vi "Test2_R_S.vi"() -> ()   [LabVIEW 2023, in "R_S.lvlib"]
uses:
  R_S.lvlib
panel:
  out "error out":errorcluster
  in  "VISA_CMD":string="SYST:PRES"
  in  "VISA in":refnum<visa-resource-name>="TCPIP::Vince_Wu-NB::inst0::INSTR"
  # "SG IP : TCPIP::192.168.88.12::hislip0::INSTR\nSA IP :  TCPIP::Vince_Wu-NB::inst0::INSTR"
  # "TCPIP::Vince_Wu-NB::inst0::INSTR"
  # "*IDN?"
  # "FETCh:WLAN:MEAS:MEValuation:TRACe:EVMagnitude:SYMBol:AVERage?"
  # "SYST:ERR?"
  # "SOUR:GPRF:GEN:RFS:LEV -20"
  # "FETCh:BURSt:ALL:FORMatted?"
  # "FETCh:BURSt:PPDU:EVM:ALL:AVERage?\nFETCh:WLAN:MEAS:MEValuation:TRACe:EVMagnitude:SYMBol:AVERage?"
  # "FETCh:BURSt:PPDU:EVM:ALL:AVERage?"
  # "FETC:BURS:ALL:FORM?"
  # "FETCh:BURSt:ALL:FORMatted?"
  # "setSA\nINIT:BLOC:CONT OFF,'Group 1'\nINIT:BLOC:IMM\nDISP:TRAC:Y:RLEV -10dBm"
  # "setPower\nSOUR:GPRF:GEN:RFS:LEV -15\n\nSOUR:GPRF:GEN:STAT ON"
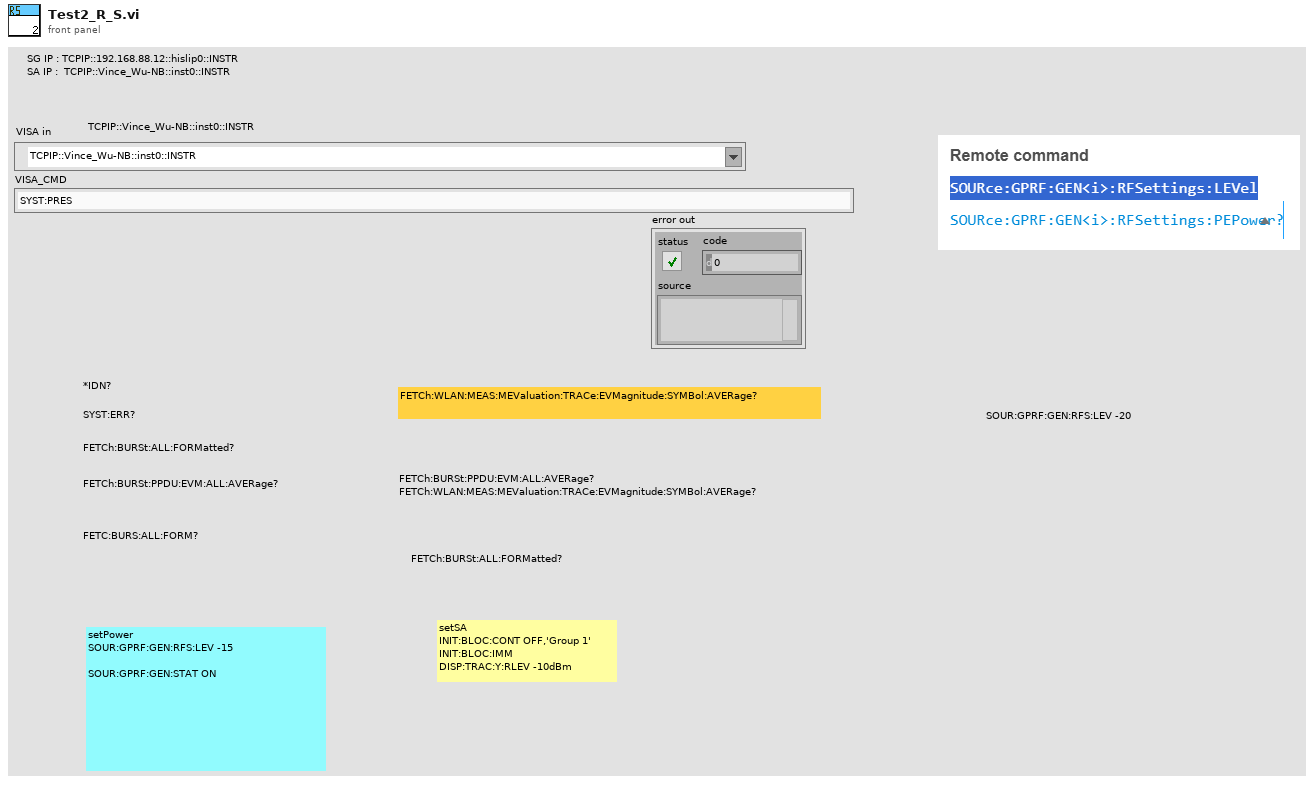
[diagram p1: front panel]
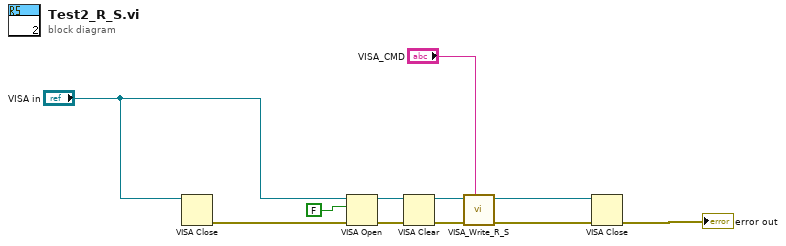
[diagram p0: block diagram]
diagram:
  n1 = VISA Close(VISA resource name="VISA in") -> (error out=w7:errorcluster)  [unwired: 1 in]
  n2 = VISA Open(duplicate session (F)=FALSE, error in (no error)=w7, VISA resource name="VISA in") -> (VISA resource name=w8:refnum<visa-resource-name>, error out=w9:errorcluster)  [unwired: 2 in]
  n3 = VISA Clear(VISA resource name=w8, error in (no error)=w9) -> (VISA resource name out=w5:refnum<visa-resource-name>, error out=w6:errorcluster)
  n4 = call "VISA_Write_R_S.vi"("VISA CMD"="VISA_CMD", "error in"=w6, "VISA in"=w5) -> ("error out"=w3:errorcluster, "VISA out"=w1:refnum<visa-resource-name>)  [unwired: 7 in]
  n5 = VISA Close(VISA resource name=w1, error in (no error)=w3) -> (error out=→"error out":errorcluster)
